vi "CHD_DRIVE_GLOBALS.vi"() -> ()   [LabVIEW 2019]
uses:
  <vilib>/Rock Robotics/WPI/ThirdParty/JAS_Junk/TrajLib/TypeDef/CHASSIS_SPEEDS.ctl
  <vilib>/Rock Robotics/WPI/ThirdParty/JAS_Junk/TrajLib/TypeDef/DIFF_DRIVE_KINEMATICS.ctl
  <vilib>/Rock Robotics/WPI/ThirdParty/JAS_Junk/TrajLib/Trajectory_Library.lvlib
panel:
  out "MotorSpeeds_MperSec":dbl[](array[numeric]) format="%17.2f"
  out "MotorDistances_M":dbl[](array[numeric]) format="%17.2f"
  out "MotorSpeedDmd_MperSec":dbl[](array[numeric]) format="%17.3f"
  out "Closed Loop Ctrl":bool
  out "Orientation_Angle_Demand_Radians":dbl format="%17.2f"
  out "Adjusted Chassis Dmd":T1 {"vOmega" format="%10.3f"; "vY" format="%10.3f"; "vX" format="%10.3f"}
  out "DIFF_DRIVE_KINEMATICS":T2 {"TrackWidth_Meters" format="%20.4f"}
  out "Swerve Chassis Speed":T1 {"vOmega" format="%10.3f"; "vY" format="%10.3f"; "vX" format="%10.3f"}
  out "GyroHeading_Radians":dbl format="%17.2f"
  out "Mod Wheel Speed Err":dbl[](array[numeric]) format="%17.3f"
  out "Mod Wheel Out":dbl[](array[numeric]) format="%17.3f"
  out "Orientation Correct CO":dbl format="%17.3f"
  out "Orientation Angle Error_Rad":dbl format="%17.3f"
  # "DIAGNOSTIC\nDATA"
  # "Overall Chassis Dmd\nafter orientation correction"
  # "Module Drive\nSpeed"
  # "Orientation Correction data"
  # "Sensor Readings"
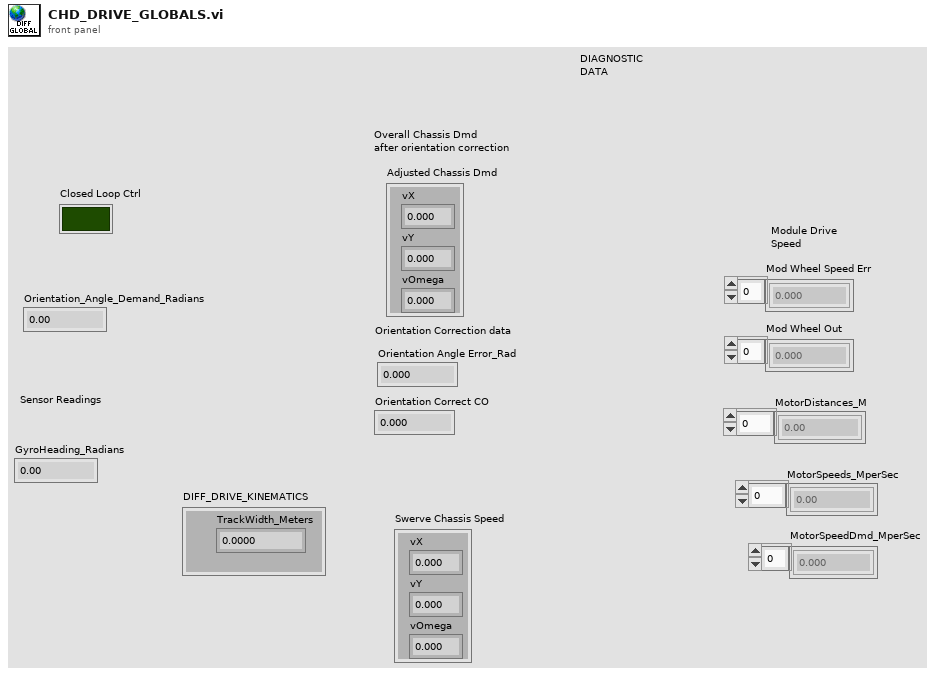
[diagram p1: front panel]
types:
  T1 = typedef "Trajectory_Library.lvlib/CHASSIS_SPEEDS.ctl" = cluster{"vX":dbl, "vY":dbl, "vOmega":dbl}
  T2 = typedef "Trajectory_Library.lvlib/DIFF_DRIVE_KINEMATICS.ctl" = cluster{"TrackWidth_Meters":dbl}
diagram:
